vi "createConfigCollection.vi"(9 "Current Config":refnum<class "Attribute.Config.lvclass">, 11 "New Config":refnum<class "Attribute.Config.lvclass">) -> (3 "Collection":refnum<class "Attribute.Config.lvclass">)   [LabVIEW 2013, in "SMO.lvclass"]
uses:
  SMO.lvclass
  Support/Attribute.Config/Attribute.Config.lvclass
  Support/Attribute.Config/Attribute.Config.lvclass/Attribute.Config.ctl
  <vilib>/LabVIEW Open Source Project/Configuration Manager/Manager/ConfigManager.lvclass
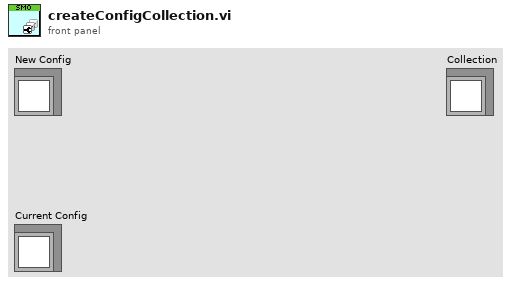
[diagram p1: front panel]
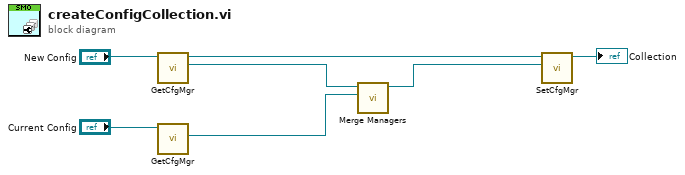
[diagram p0: block diagram]
diagram:
  n1 = call "GetCfgMgr.vi"("Attribute.Config in"="New Config") -> ("CfgMgr"=w3:refnum<class "ConfigManager.lvclass">, "Attribute.Config out"=w5:refnum<class "Attribute.Config.lvclass">)  [unwired: 9 in]
  n2 = call "GetCfgMgr.vi"("Attribute.Config in"="Current Config") -> ("CfgMgr"=w2:refnum<class "ConfigManager.lvclass">)  [unwired: 9 in, 1 out]
  n3 = call <vilib>:"Merge Managers.vi"("ConfigManager B"=w2, "ConfigManager A"=w3) -> ("ConfigManagerCollection"=w1:refnum<class "ConfigManagerCollection.lvclass">)  [unwired: 9 in]
  n4 = call "SetCfgMgr.vi"("CfgMgr"=w1, "Attribute.Config in"=w5) -> ("Attribute.Config out"=→"Collection":refnum<class "Attribute.Config.lvclass">)  [unwired: 9 in]
